vi "exnSpectralBlock spectral measurements RMS DDT.vi"(0 "Signals":dynamicdata(graph), 5 "Restart Averaging":bool, 7 "View":T2, 9 "Spectrum Window":u16, 11 "error in (no error)":errorcluster, 12 "Spectrum Averaging Parameters":T1={"averaging mode"=0, "weighting mode"=1, "number of averages"=10} {"averaging mode" items=["No averaging", "Vector averaging", "RMS averaging", "Peak hold"]; "weighting mode" items=["Linear", "Exponential"]}, 14 "All Spectra":bool) -> (4 "Measurement Output":dynamicdata(graph), 6 "averaging done":bool, 10 "Phase":dynamicdata(graph), 15 "error out":errorcluster)   [LabVIEW 2017]
uses:
  <vilib>/measure/NI_MAPro.lvlib
panel:
  in  "measurement":string="FFT - (RMS)"
  in  "string":string=" Phase"
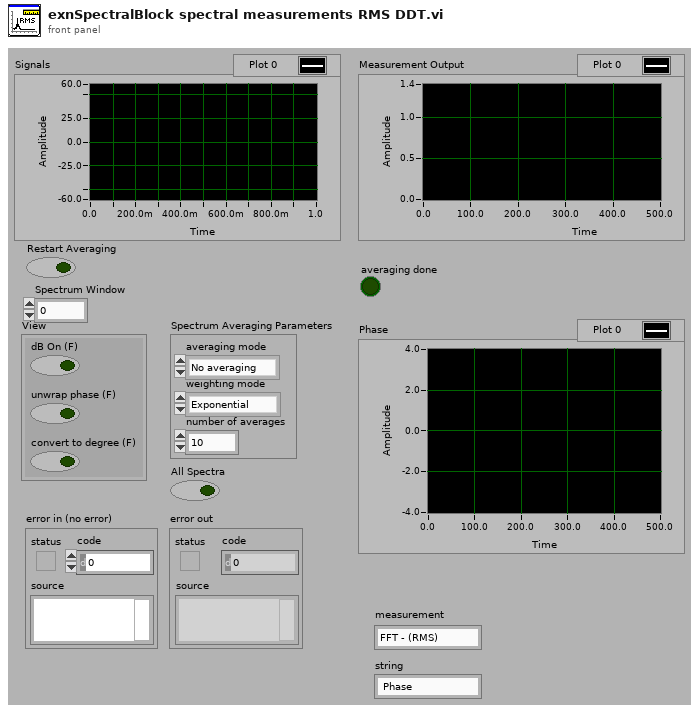
[diagram p1: front panel]
types:
  T1 = cluster{"averaging mode":u16, "weighting mode":u16, "number of averages":u32}
  T2 = cluster{"dB On (F)":bool, "unwrap phase (F)":bool, "convert to degree (F)":bool}
  T3 = enum16{"None ", "Hanning", "Hamming", "Blackman-Harris", "Exact Blackman", "Blackman", "Flat Top", "4 Term B-Harris ", "7 Term B-Harris", "Low Sidelobe"}
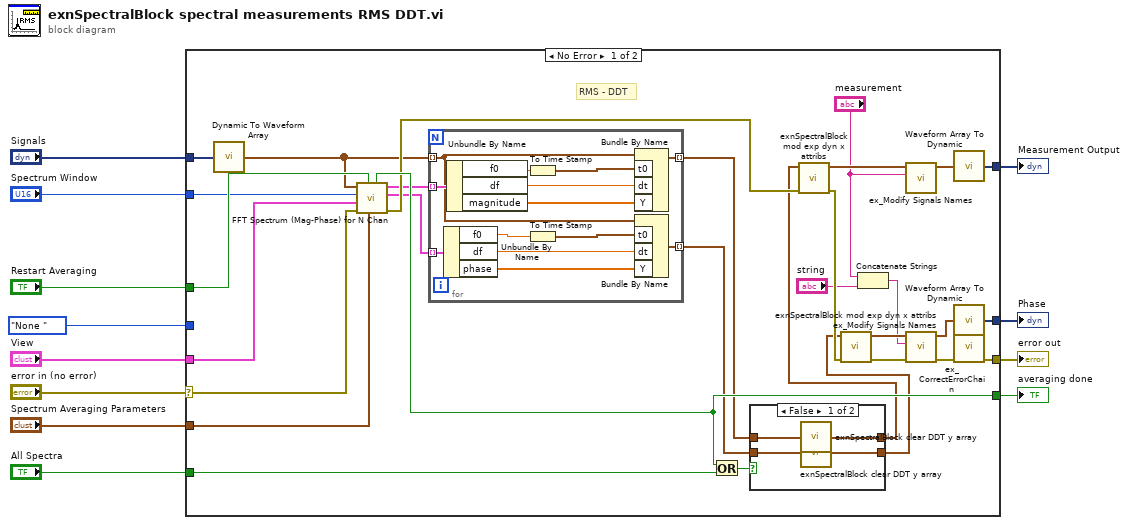
[diagram p0: block diagram]
diagram:
  n1 = case shown="No Error" "error in (no error)" {
    selector: "error in (no error)" -> [w16 w62]
    tunnel: [w42 _] -> w12
    tunnel: [w41 _] -> w11
    tunnel: [w40 _] -> w10
    tunnel: "All Spectra" -> [w39 _]
    tunnel: "Spectrum Averaging Parameters" -> [w38 _]
    tunnel: "Restart Averaging" -> [w37 _]
    tunnel: T3."None " ("window") -> [_ _]
    tunnel: "Spectrum Window" -> [w17 _]
    tunnel: "View" -> [w35 _]
    tunnel: "Signals" -> [w33 _]
    tunnel: [w32 w62] -> w3
    frame No Error {
      # "RMS - DDT"
      n2 = call <vilib>:"Dynamic To Waveform Array.vi"("Input"=w33) -> ("Output"=w18:waveform(dbl)[])  [unwired: 4 in]
      n3 = call <vilib>:"FFT Spectrum (Mag-Phase) for N Chan.vi"("averaging parameters"=w38, "restart averaging (F)"=w37, "error in (no error)"=w16, "view"=w35, "window"=w17, "time signals"=w18) -> ("error out"=w34:errorcluster, "phases"=w13:cluster{"f0":dbl, "df":dbl, "phase":dbl[]}[], "magnitudes"=w14:cluster{"f0":dbl, "df":dbl, "magnitude":dbl[]}[], "averaging done"=w40:bool)  [unwired: 1 in, 1 out]
      n4 = for {
        tunnel: w18 -> [w45] mode=indexing
        tunnel: [w52] -> w21 mode=indexing
        tunnel: w14 -> [w51] mode=indexing
        tunnel: w13 -> [w44] mode=indexing
        tunnel: [w43] -> w22 mode=indexing
        n5 = Unbundle By Name(w44) -> ("f0"=w48:dbl, "df"=w47:dbl, "phase"=w46:dbl[])
        n6 = Unbundle By Name(w51) -> ("f0"=w53:dbl, "df"=w54:dbl, "magnitude"=w55:dbl[])
        n7 = To Time Stamp(1:w53) -> (0:w50:timestamp)
        n8 = To Time Stamp(1:w48) -> (0:w49:timestamp)
        n9 = Bundle By Name(cluster=w45, "t0"=w50, "dt"=w54, "Y"=w55) -> (w52:waveform(dbl))
        n10 = Bundle By Name(cluster=w45, "t0"=w49, "dt"=w47, "Y"=w46) -> (w43:waveform(dbl))
      }
      n11 = Or(x=w40, y=w39) -> (x .or. y?=w23:bool)
      n12 = case shown="False" w23 {
        tunnel: w22 -> [w57 w60]
        tunnel: w21 -> [w59 w61]
        tunnel: [w58 w61] -> w20
        tunnel: [w56 w60] -> w19
        frame False {
          n13 = call <vilib>:"exnSpectralBlock clear DDT y array.vi"("Array In"=w59) -> ("Array Out"=w58:waveform(dbl)[])
          n14 = call <vilib>:"exnSpectralBlock clear DDT y array.vi"("Array In"=w57) -> ("Array Out"=w56:waveform(dbl)[])
        }
        frame True {
        }
      }
      n15 = call <vilib>:"exnSpectralBlock mod exp dyn x attribs.vi"("error in (no error)"=w34, "Signals in"=w20) -> ("error out"=w36:errorcluster, "Signals out"=w31:waveform(dbl)[])  [unwired: 8 in]
      n16 = call <vilib>:"exnSpectralBlock mod exp dyn x attribs.vi"("error in (no error)"=w36, "Signals in"=w19) -> ("error out"=w29:errorcluster, "Signals out"=w26:waveform(dbl)[])  [unwired: 8 in]
      n17 = Concatenate Strings("measurement", "string") -> (w24:string)
      n18 = call <vilib>:"ex_Modify Signals Names.vi"("Name Modifier"="measurement", "Array of Waveforms In"=w31) -> ("Array of Waveforms Out"=w30:waveform(dbl)[])  [unwired: 8 in, 1 out]
      n19 = call <vilib>:"ex_Modify Signals Names.vi"("error in (no error)"=w29, "Name Modifier"=w24, "Array of Waveforms In"=w26) -> ("error out"=w28:errorcluster, "Array of Waveforms Out"=w27:waveform(dbl)[])  [unwired: 7 in]
      n20 = call <vilib>:"Waveform Array To Dynamic.vi"("Input"=w30) -> ("Output"=w42:dynamicdata)  [unwired: 4 in]
      n21 = call <vilib>:"Waveform Array To Dynamic.vi"("Input"=w27) -> ("Output"=w41:dynamicdata)  [unwired: 4 in]
      n22 = call <vilib>:"ex_CorrectErrorChain.vi"("error in (no error)"=w28) -> ("error out"=w32:errorcluster)  [unwired: 10 in]
    }
    frame Error {
    }
  }
  "Phase" <- w11
  "Measurement Output" <- w12
  "averaging done" <- w10
  "error out" <- w3
